vi "BooleanNotifier Init.vi"(8 "error in (no error)":errorcluster, 10 "name (unnamed)":string) -> (0 "error out":errorcluster, 3 "BooleanNotifier out":refnum<class "BooleanNotifier.lvclass">)   [LabVIEW 2018, in "BooleanNotifier.lvclass"]
uses:
  BooleanNotifier.lvclass
  BooleanNotifier.lvclass/BooleanNotifier.ctl
panel:
  in  "BooleanNotifier in":refnum<class "BooleanNotifier.lvclass">
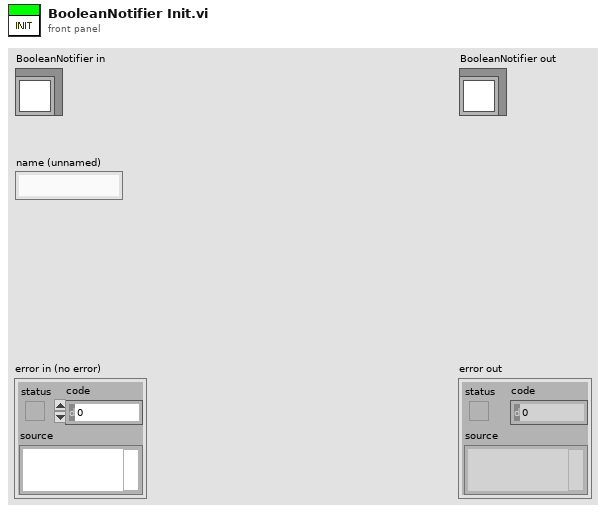
[diagram p1: front panel]
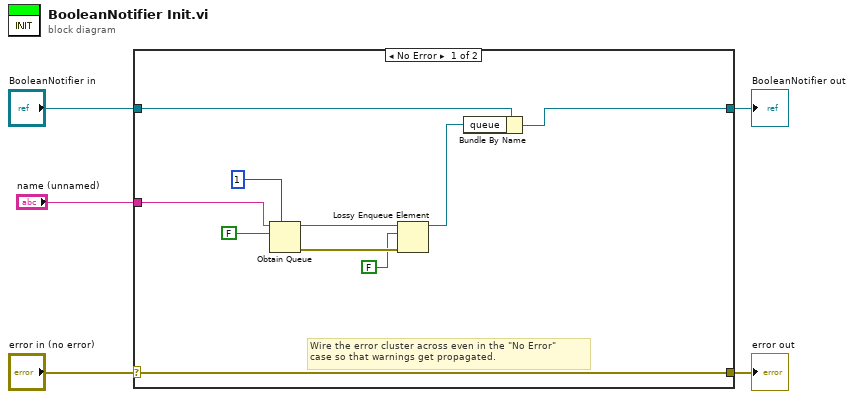
[diagram p0: block diagram]
diagram:
  n1 = case shown="No Error" "error in (no error)" {
    selector: "error in (no error)" -> [w14 w17]
    tunnel: [w14 w17] -> w4
    tunnel: [w13 w16] -> w2
    tunnel: "BooleanNotifier in" -> [w15 w16]
    tunnel: "name (unnamed)" -> [w10 _]
    frame No Error {
      # "Wire the error cluster across even in the \"No Error\"\ncase so that warnings get propagated."
      n2 = Obtain Queue(max queue size (-1, unlimited)=1, name (unnamed)=w10, element data type=FALSE) -> (queue out=w8:refnum<queue>, error out=w9:errorcluster)  [unwired: 2 in, 1 out]
      n3 = Lossy Enqueue Element(queue=w8, element=FALSE, error in (no error)=w9) -> (queue out=w7:refnum<queue>)  [unwired: 3 out]
      n4 = Bundle By Name(cluster=w15, "queue"=w7) -> (w13:refnum<class "BooleanNotifier.lvclass">)
    }
    frame Error {
    }
  }
  "error out" <- w4
  "BooleanNotifier out" <- w2
